vi "FindValueInArrayFromCluster.vi"(1 "Value":dbl, 2 "Correction":cluster{dbl, dbl}[](array[cluster])) -> (0 "Output":dbl)   [LabVIEW 2010]
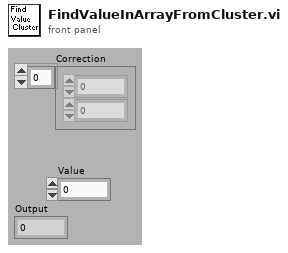
[diagram p1: front panel]
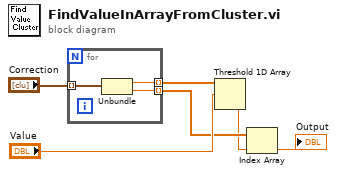
[diagram p0: block diagram]
diagram:
  n1 = for {
    tunnel: "Correction" -> [w9] mode=indexing
    tunnel: [w8] -> w5 mode=indexing
    tunnel: [w7] -> w3 mode=indexing
    n2 = Unbundle(w9) -> (w8:dbl, w7:dbl)
  }
  n3 = Threshold 1D Array(2:"Value", 3:w5) -> (0:w2:dbl)  [unwired: 1 in]
  n4 = Index Array(array=w3, index=w2) -> (element=→"Output":dbl)
